vi "Convert Node Result to Test Suite - Assertions with Properties - Same Number of Properties.vi"() -> ()   [LabVIEW 2013, in "JUnit Conversion Tests.lvlib"]
uses:
  JUnit Conversion Tests.lvlib
  <vilib>/addons/_JKI Toolkits/Caraya/classes/Test Result/Node Results (Extended).ctl
  <vilib>/addons/_JKI Toolkits/Caraya/classes/Test Result/Test Node (Extended).ctl
  <vilib>/addons/_JKI Toolkits/Caraya/classes/Test Result/Test Registration Data.ctl
  <vilib>/addons/_JKI Toolkits/Caraya/classes/Test Result/Assert Event Data (Extended).ctl
  <vilib>/addons/_JKI Toolkits/Caraya/classes/MsgSerializer/MsgSerializer.lvclass
  JUnit XML/Test Suite/Test Suite.lvclass/Test Suite.ctl
  JUnit XML/Test Suite/Read Properties.vi
  <vilib>/addons/_JKI Toolkits/Caraya/classes/Assert/Assert Equal Value_Variant.vi
  JUnit XML/Property/Property.lvclass
  <vilib>/addons/_JKI Toolkits/Caraya/classes/Assert/Assert.lvclass
  <vilib>/addons/_JKI Toolkits/Caraya/classes/Test/Test.lvclass
  JUnit Conversion/JUnit Conversion.lvlib
  <vilib>/addons/_JKI Toolkits/Caraya/classes/Test Result/Test Result.lvclass
  JUnit XML/Test Suite/Test Suite.lvclass
panel:
  out "error out":errorcluster
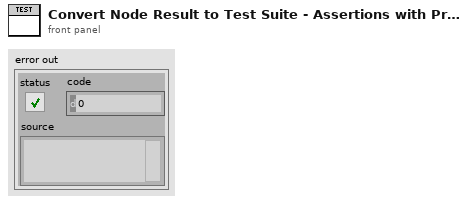
[diagram p1: front panel]
types:
  T1 = typedef "Caraya.lvlib/Test Result.lvclass/Assert Event Data (Extended).ctl" = cluster{"name":string, "passed":bool, "call-chain":string[], "test-error":errorcluster, "timestamp":timestamp, "assert-id":string, "test-id":string, "time":dbl, "message":string, "properties":variant, "measurements":variant, "user-defined":variant}
  T2 = typedef "Caraya.lvlib/Test Result.lvclass/Node Results (Extended).ctl" = cluster{"Test Node":T3, "Assertions":T1[]}
  T3 = typedef "Caraya.lvlib/Test Result.lvclass/Test Node (Extended).ctl" = cluster{"Test Registration":T4, "Defined":bool, "Passed":bool, "properties":variant}
  T4 = typedef "Caraya.lvlib/Test Result.lvclass/Test Registration Data.ctl" = cluster{"Name":string, "Call Chain":string[], "Time Stamp":timestamp, "Test ID":string, "Caller ID":string}
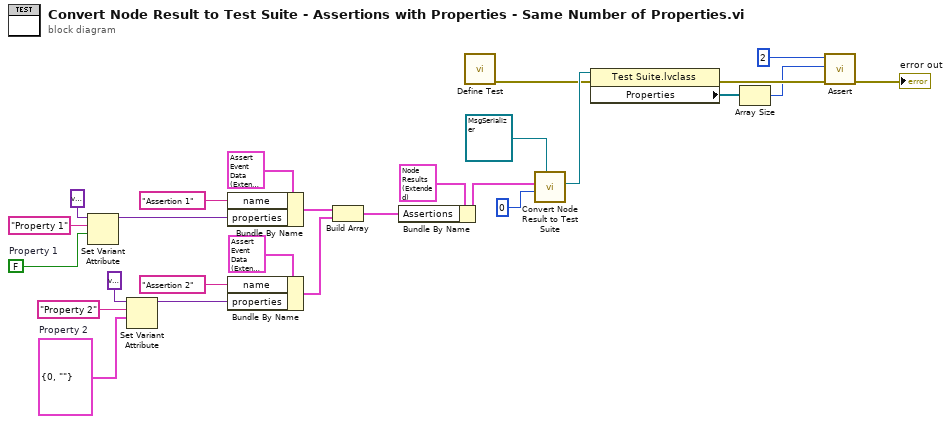
[diagram p0: block diagram]
diagram:
  w7 = cluster{"Numeric":i32, "String":string} {"Numeric"=0, "String"=""}  # Property 2
  w4 = FALSE  # Property 1
  n1 = Set Variant Attribute(Variant=variant ("variant"), name="Property 1", value=w4) -> (Variant out=w5:variant)  [unwired: 1 in, 2 out]
  n2 = Set Variant Attribute(Variant=variant ("variant"), name="Property 2", value=w7) -> (Variant out=w8:variant)  [unwired: 1 in, 2 out]
  n3 = Bundle By Name(cluster=T1 {"name"="", "passed"=FALSE, "call-chain"=[], "test-error"={"status"=FALSE, "code"=0, "source"=""}, "timestamp"=timestamp(0 s since 1904-01-01), "assert-id"="", "test-id"="", "time"=0.0, "message"="", "properties"=variant, "measurements"=variant, "user-defined"=variant} ("Assert Event Data"), "name"="Assertion 1", "properties"=w5) -> (w18:T1)
  n4 = Bundle By Name(cluster=T1 {"name"="", "passed"=FALSE, "call-chain"=[], "test-error"={"status"=FALSE, "code"=0, "source"=""}, "timestamp"=timestamp(0 s since 1904-01-01), "assert-id"="", "test-id"="", "time"=0.0, "message"="", "properties"=variant, "measurements"=variant, "user-defined"=variant} ("Assert Event Data"), "name"="Assertion 2", "properties"=w8) -> (w13:T1)
  n5 = Build Array(w18, w13) -> (w17:T1[])
  n6 = Bundle By Name(cluster=T2 {"Test Node"={"Test Registration"={"Name"="", "Call Chain"=[], "Time Stamp"=timestamp(0 s since 1904-01-01), "Test ID"="", "Caller ID"=""}, "Defined"=FALSE, "Passed"=FALSE, "properties"=variant}, "Assertions"=[]} ("Node Result"), "Assertions"=w17) -> (w21:T2)
  n7 = call <vilib>:"Define Test.vi"() -> ("error out"=w25:errorcluster)  [unwired: 10 in, 1 out]
  n8 = call "Convert Node Result to Test Suite.vi"("MsgSerializer"=refnum<class "MsgSerializer.lvclass"> refnum, "ID"=0, "Node Result"=w21) -> ("Test Suite"=w26:refnum<class "Test Suite.lvclass">)  [unwired: 8 in]
  n9 = property class="Test Suite.lvclass"(reference=w26, error in=w25) -> (error out=w12:errorcluster, "Properties"=w10:refnum<class "Property.lvclass">[])  [unwired: 1 out]
  n10 = Array Size(array=w10) -> (size(s)=w9:i32)
  n11 = call-poly <vilib>:"Assert.vi"("error in (no error)"=w12, "Y"=w9, "X"=2 ("size(s)")) -> ("error out"=→"error out":errorcluster)  [unwired: 7 in, 1 out]
